vi "destroy.vi"(8 "error in)":errorcluster, 10 "MQTT events":T1, 11 "MQTT Context":u64) -> (0 "error out":errorcluster)   [LabVIEW 2013, in "MQTT.lvlib"]
uses:
  MQTT.lvlib
  events.ctl
  subMsg.ctl
  statusMsg.ctl
  msgAck.ctl
  paho-mqtt3a.dll
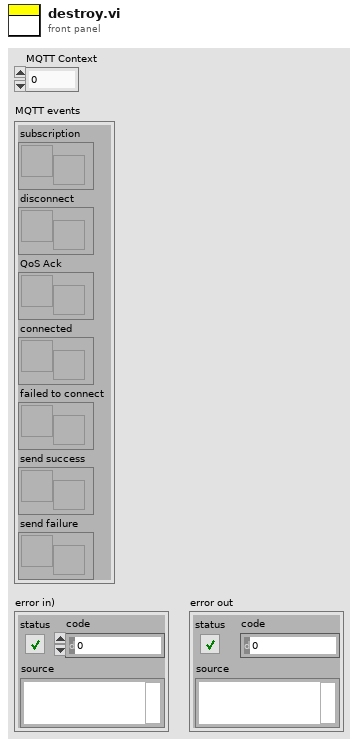
[diagram p1: front panel]
types:
  T1 = typedef "MQTT.lvlib/events.ctl" = cluster{"subscription":refnum<user-event>, "disconnect":refnum<user-event>, "QoS Ack":refnum<user-event>, "connected":refnum<user-event>, "failed to connect":refnum<user-event>, "send success":refnum<user-event>, "send failure":refnum<user-event>}
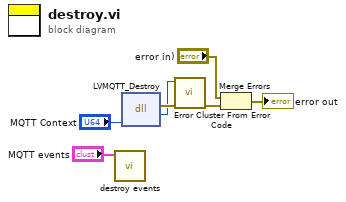
[diagram p0: block diagram]
diagram:
  n1 = call "destroy events.vi"("MQTT events"="MQTT events") -> ()  [unwired: 11 in]
  n2 = dll-call lib="C:/Users/Daniel/Documents/MQTT/LVMQTT/paho-mqtt3a.dll" fn="LVMQTT_Destroy"("lvctx"="MQTT Context") -> (error out=w6:errorcluster, "return type"=w4:i32)  [unwired: 4 in, 1 out]
  n3 = call <vilib>:"Error Cluster From Error Code.vi"("error in (no error)"=w6, "error code (0)"=w4) -> ("error out"=w5:errorcluster)  [unwired: 7 in]
  n4 = Merge Errors("error in)", w5) -> (→"error out":errorcluster)
